vi "calculateBissectriz.vi"(8 "error in (no error)":errorcluster, 9 "Array 2":dbl[](array[numeric]), 10 "Array":dbl[](array[numeric]), 11 "Utilities in":refnum<class "Utilities.lvclass">) -> (0 "error out":errorcluster, 2 "Bissectriz":dbl[](array[numeric]), 3 "Utilities out":refnum<class "Utilities.lvclass">)   [LabVIEW 2023, in "Utilities.lvclass"]
uses:
  Utilities.lvclass
  <vilib>/Analysis/baseanly.llb/Unit Vector (DBL).vi
  <vilib>/Analysis/coordinate.llb/2D Cartesian Coordinate Rotation (Scalar).vi
  <vilib>/Analysis/NI_AALPro.lvlib
  <vilib>/Analysis/NI_AALBase.lvlib
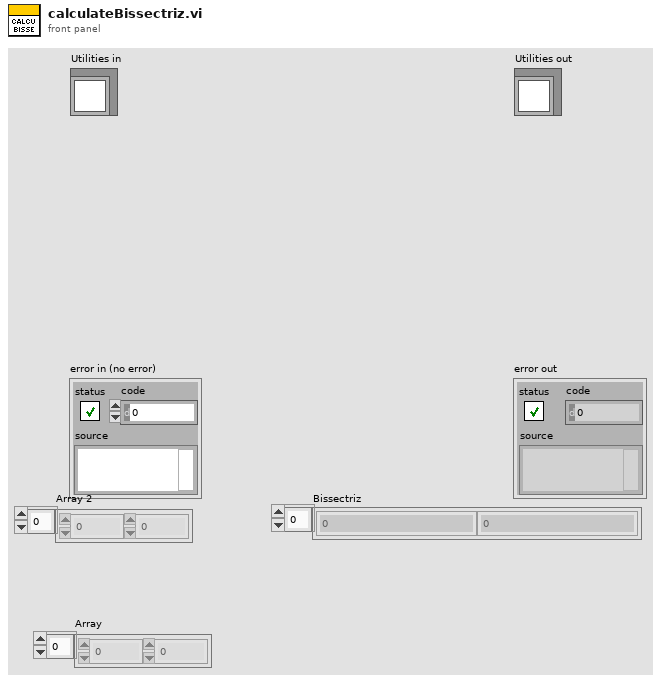
[diagram p1: front panel]
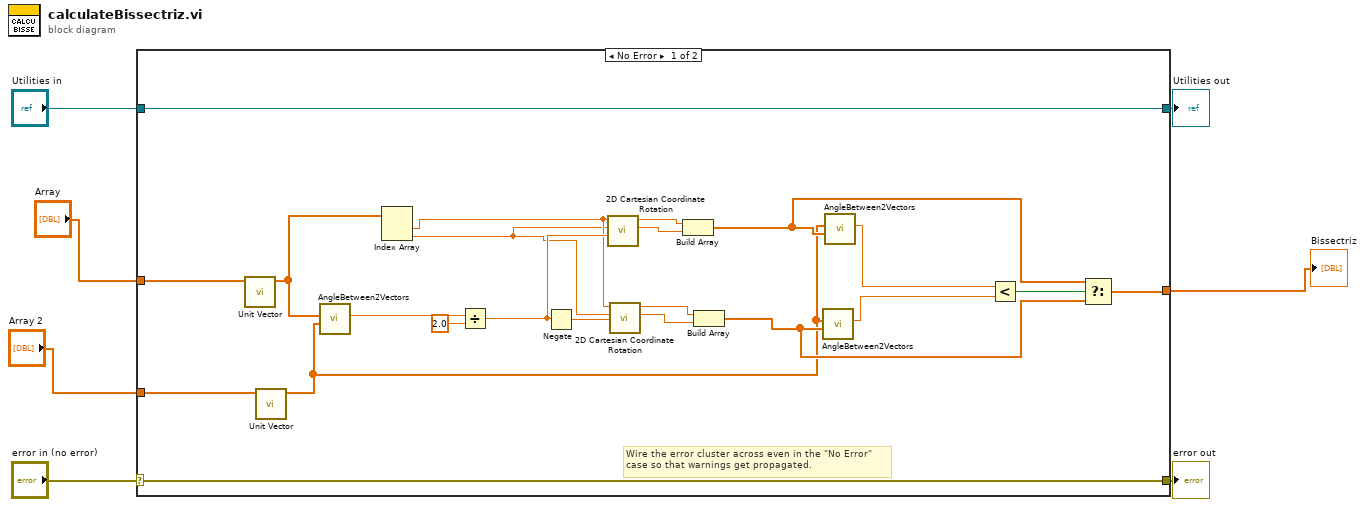
[diagram p0: block diagram]
diagram:
  n1 = case shown="No Error" "error in (no error)" {
    selector: "error in (no error)" -> [w28 w31]
    tunnel: [w28 w31] -> w6
    tunnel: [w29 w30] -> w4
    tunnel: "Utilities in" -> [w29 w30]
    tunnel: "Array" -> [w10 _]
    tunnel: "Array 2" -> [w9 _]
    tunnel: [w8 _] -> w1
    frame No Error {
      # "Wire the error cluster across even in the \"No Error\"\ncase so that warnings get propagated."
      n2 = call-poly <vilib>:"Unit Vector.vi"("Input Vector"=w10) -> ("Unit Vector"=w12:dbl[])  [unwired: 8 in, 2 out]
      n3 = call-poly <vilib>:"Unit Vector.vi"("Input Vector"=w9) -> ("Unit Vector"=w11:dbl[])  [unwired: 8 in, 2 out]
      n4 = call "AngleBetween2Vectors.vi"("Array 1"=w11, "Array 2"=w12) -> ("angleInRadians(default)"=w27:dbl)  [unwired: 6 in, 3 out]
      n5 = Index Array(array=w12) -> (element #1=w23:dbl, element #2=w22:dbl)  [unwired: 2 in]
      n6 = Divide(x=w27, y=2.0) -> (x/y=w24:dbl)
      n7 = Negate(x=w24) -> (-x=w25:dbl)
      n8 = call-poly <vilib>:"2D Cartesian Coordinate Rotation.vi"("theta"=w24, "y"=w22, "x"=w23) -> ("y out"=w20:dbl, "x out"=w21:dbl)  [unwired: 6 in, 1 out]
      n9 = call-poly <vilib>:"2D Cartesian Coordinate Rotation.vi"("theta"=w25, "y"=w22, "x"=w23) -> ("y out"=w18:dbl, "x out"=w19:dbl)  [unwired: 6 in, 1 out]
      n10 = Build Array(w21, w20) -> (w14:dbl[])
      n11 = Build Array(w19, w18) -> (w13:dbl[])
      n12 = call "AngleBetween2Vectors.vi"("Array 1"=w13, "Array 2"=w11) -> ("angleInRadians(default)"=w16:dbl)  [unwired: 6 in, 3 out]
      n13 = call "AngleBetween2Vectors.vi"("Array 1"=w14, "Array 2"=w11) -> ("angleInRadians(default)"=w17:dbl)  [unwired: 6 in, 3 out]
      n14 = Less?(x=w17, y=w16) -> (x < y?=w15:bool)
      n15 = Select(t=w14, s=w15, f=w13) -> (s? t:f=w8:dbl[])
    }
    frame Error {
    }
  }
  "error out" <- w6
  "Utilities out" <- w4
  "Bissectriz" <- w1
